vi "Get DDG Pulse.vi"(7 "Width":dbl, 8 "error in (no error)":errorcluster, 9 "Delay":dbl, 10 "resolution":dbl, 11 "wid":dbl) -> (0 "error out":errorcluster, 1 "Delay out":dbl, 3 "function return":u32, 5 "Width out":dbl)   [LabVIEW 2014, in "atmcd32d.lvlib"]
doc: "unsigned int WINAPI GetDDGPulse(double wid, double resolution, double * Delay, double * Width);"
uses:
  atmcd32d.lvlib
  atmcd32d.dll
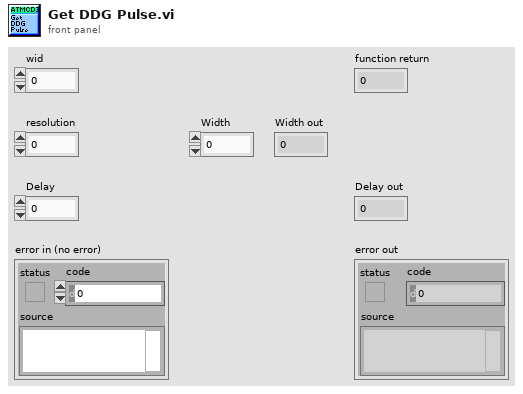
[diagram p1: front panel]
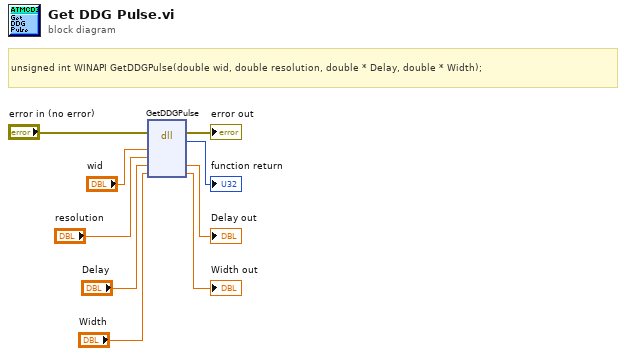
[diagram p0: block diagram]
diagram:
  # "unsigned int WINAPI GetDDGPulse(double wid, double resolution, double * Delay, double * Width);"
  n1 = dll-call lib="C:/Users/Bakir/Documents/Lambda2-Testing/lib/Andorlib/atmcd32d.*" fn="GetDDGPulse"(error in="error in (no error)", "wid"="wid", "resolution"="resolution", "Delay"="Delay", "Width"="Width") -> (error out=→"error out":errorcluster, →"function return":u32, "Delay"=→"Delay out":dbl, "Width"=→"Width out":dbl)  [unwired: 4 in, 1 out]
